vi "Config Database Top level.vi"(8 "error in (no error)":errorcluster) -> (0 "error out":errorcluster)   [LabVIEW 2013, in "ConfigDBLib.lvlib"]
doc: "Config Database is used to update the balance after Deposit, Withdrawal and Fast Casg $ 50 and Maintain the account info."
uses:
  ConfigDBLib.lvlib
  Private Controls/Queue Driver Control_Config DB.ctl
  Private Controls/Balance Update.ctl
  MainVI/TopLevelController/ToplevelControllerLibrary.lvlib
panel:
  # "Config Database is used to update the balance after Deposit, Withdrawal and Fast Casg $ 50 and Maintain the account info."
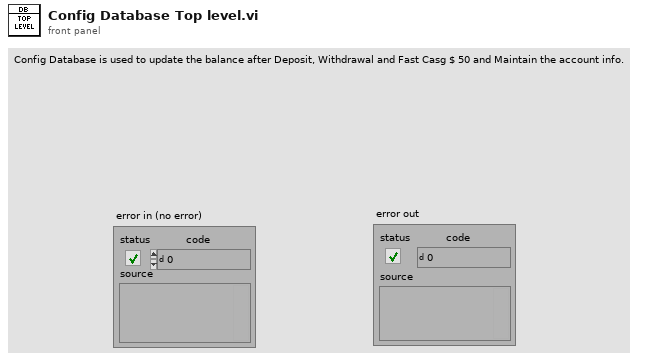
[diagram p1: front panel]
types:
  T1 = enum16{"Create Event", "Generate Event", "Destroy Event"}
  T2 = typedef "ConfigDBLib.lvlib/Queue Driver Control_Config DB.ctl" = enum16{"Init", "Enqueue", "Dequeue", "ReleaseQueue", "Exit"}
  T3 = typedef "ConfigDBLib.lvlib/Balance Update.ctl" = enum16{"Balance", "Deposit", "Withdrawal", "FastCash"}
  T4 = enum16{"Init", "Enqueue", "Dequeue", "ReleaseQueue", "Exit"}
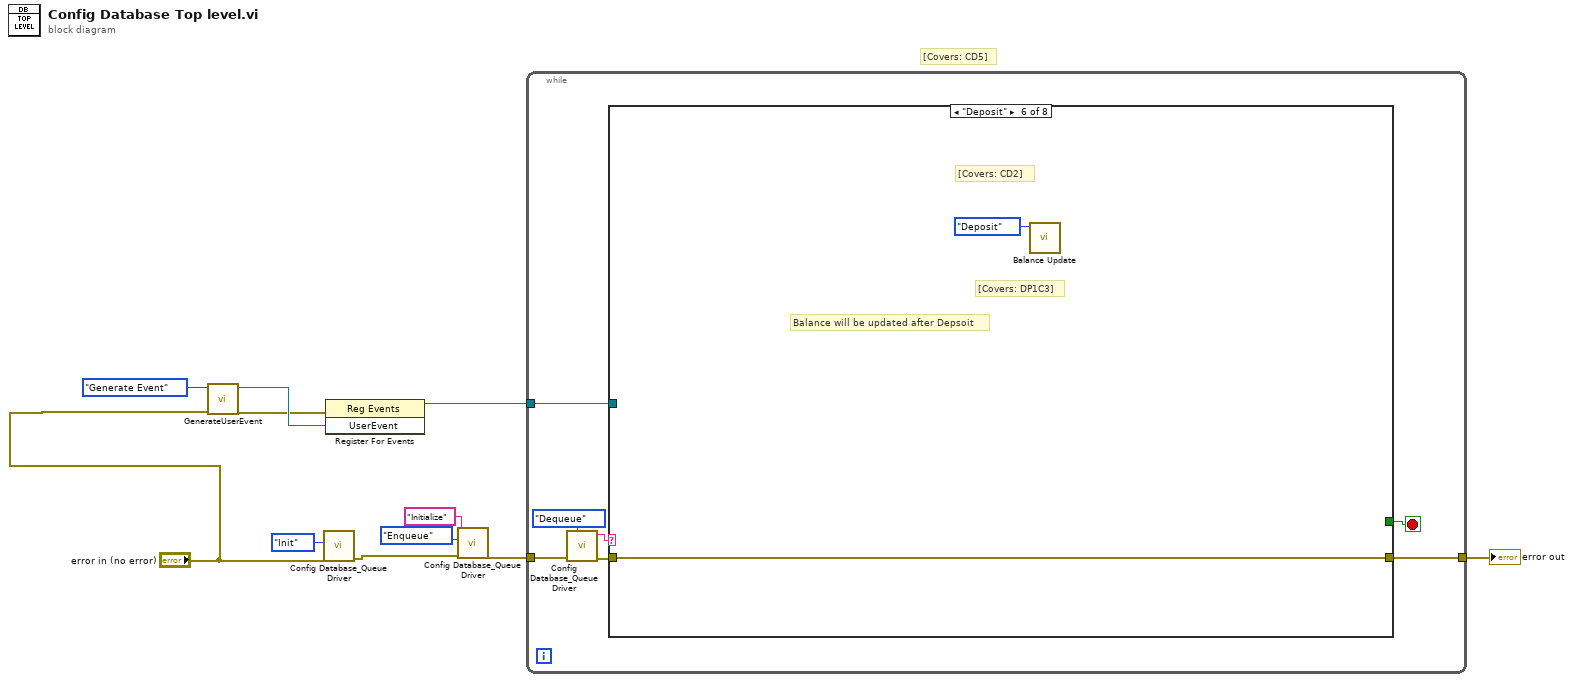
[diagram p0: block diagram]
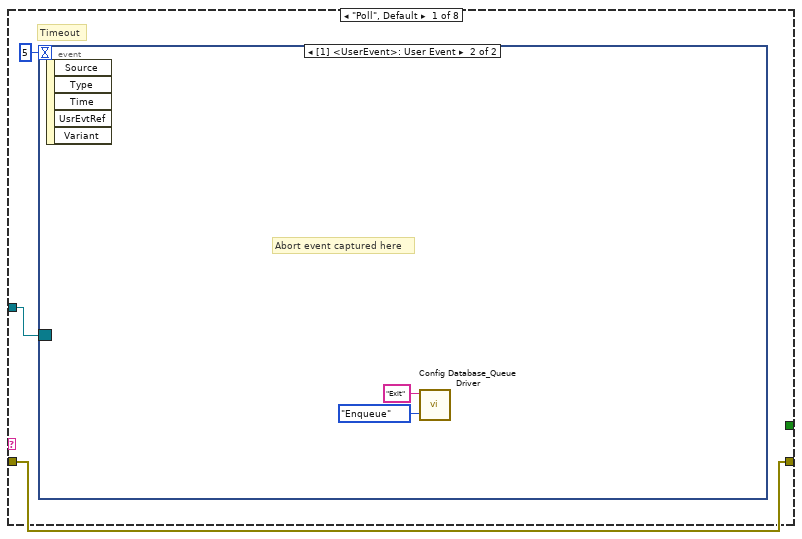
[diagram p2: hidden frame]
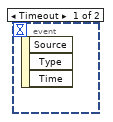
[diagram p3: hidden frame]
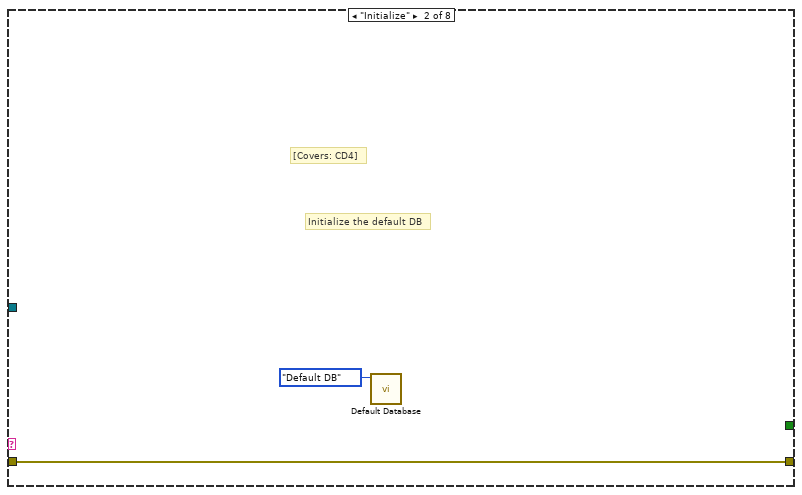
[diagram p4: hidden frame]
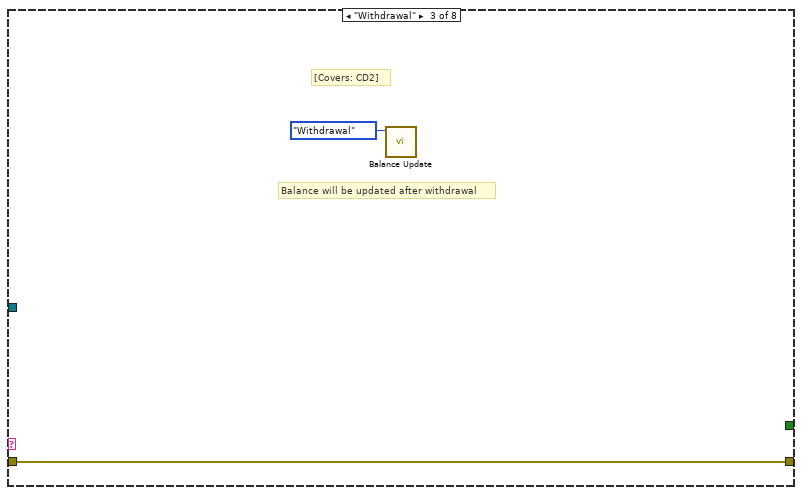
[diagram p5: hidden frame]
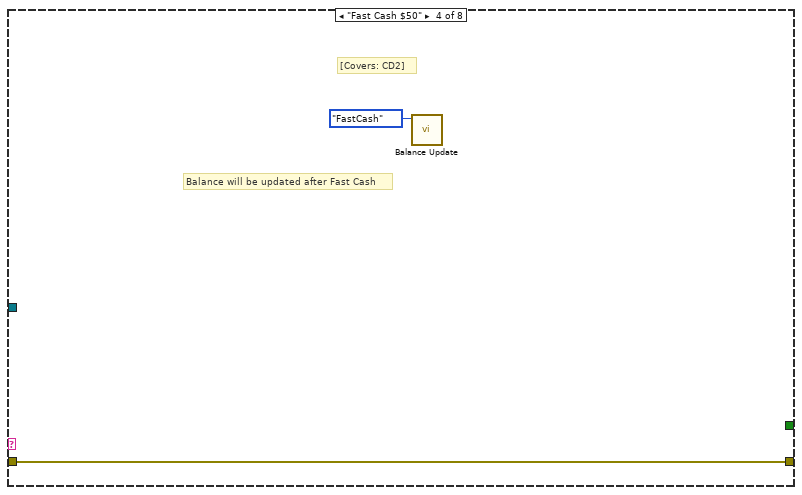
[diagram p6: hidden frame]
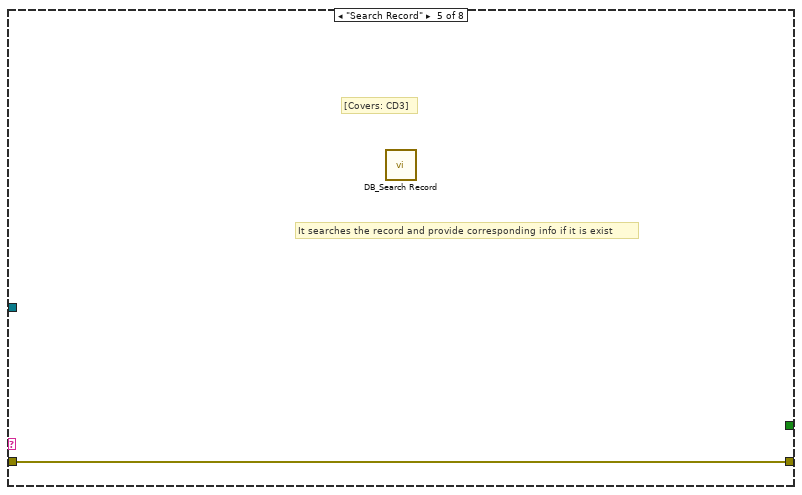
[diagram p7: hidden frame]
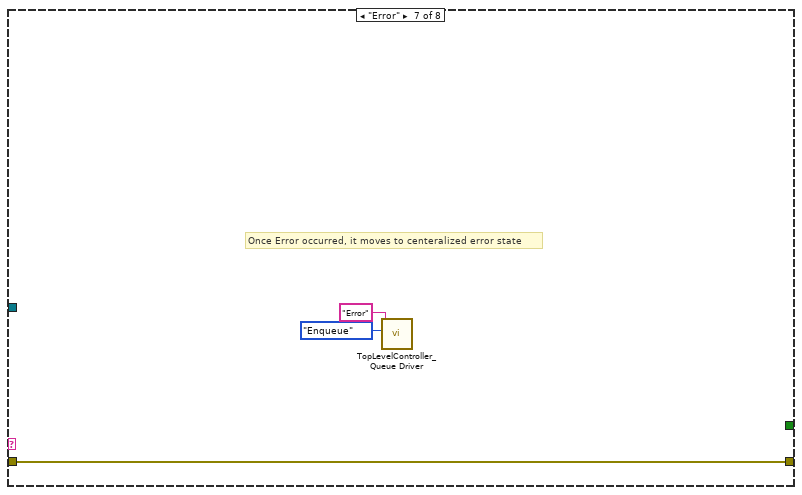
[diagram p8: hidden frame]
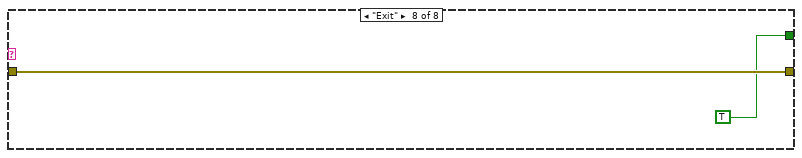
[diagram p9: hidden frame]
diagram:
  # "[Covers: CD5]"
  n1 = call "GenerateUserEvent.vi"("error in (no error)"="error in (no error)", "Event Actions"=T1."Generate Event") -> ("error out"=w3:errorcluster, "UserEvent"=w4:refnum<user-event>)  [unwired: 8 in]
  n2 = call "Config Database_Queue Driver.vi"("error in (no error)"="error in (no error)", "Enum"=Queue_Driver_Control_Config_DB."Init") -> ("error out"=w8:errorcluster)  [unwired: 8 in, 1 out]
  n3 = register-events(error in=w3, w4) -> (reference out=w2:refnum<event-registration>)  [unwired: 1 in, 1 out]
  n4 = call "Config Database_Queue Driver.vi"("error in (no error)"=w8, "Enum"=Queue_Driver_Control_Config_DB."Enqueue", "EnQ"="Initialize") -> ("error out"=w7:errorcluster)  [unwired: 7 in, 1 out]
  n5 = while {
    tunnel: w7 -> [w16]
    tunnel: [w18] -> w11
    tunnel: w2 -> [w12]
    stop <- w17 stop-if-true
    n6 = call "Config Database_Queue Driver.vi"("error in (no error)"=w16, "Enum"=Queue_Driver_Control_Config_DB."Dequeue") -> ("error out"=w13:errorcluster, "DeQ"=w14:string)  [unwired: 8 in]
    n7 = case shown="\"Deposit\"" w14 {
      tunnel: [w20 w25 w27 w29 w30 w32 w35 w37] -> w18
      tunnel: w13 -> [w20 w25 w27 w29 w30 w32 w35 w37]
      tunnel: [_ _ _ _ _ _ _ TRUE] -> w17
      tunnel: w12 -> [w19 _ _ _ _ _ _ _]
      frame "Poll", Default {
        # "Timeout"
        n8 = event shown="[1] <UserEvent>: User Event" {
          selector: w19 -> [_ _]
          dyn-events: _ -> [_ _]
          timeout: 5 -> [_ _]
          event Timeout {
            n9 = event-data() -> ()  [unwired: 1 in, 3 out]
          }
          event User Event {
            # "Abort event captured here"
            n10 = event-data() -> ()  [unwired: 1 in, 5 out]
            n11 = call "Config Database_Queue Driver.vi"("Enum"=Queue_Driver_Control_Config_DB."Enqueue", "EnQ"="Exit") -> ()  [unwired: 8 in, 2 out]
          }
        }
      }
      frame "Initialize" {
        # "Initialize the default DB"
        # "[Covers: CD4]"
        n12 = call "Default Database.vi"("Enum"=enum16{"", "Default DB", "Actual DB"}."Default DB") -> ()  [unwired: 10 in, 1 out]
      }
      frame "Withdrawal" {
        # "Balance will be updated after withdrawal"
        # "[Covers: CD2]"
        n13 = call "Balance Update.vi"("Bal.Update"=Balance_Update."Withdrawal") -> ()  [unwired: 10 in, 1 out]
      }
      frame "Fast Cash $50" {
        # "Balance will be updated after Fast Cash"
        # "[Covers: CD2]"
        n14 = call "Balance Update.vi"("Bal.Update"=Balance_Update."FastCash") -> ()  [unwired: 10 in, 1 out]
      }
      frame "Search Record" {
        # "It searches the record and provide corresponding info if it is exist"
        # "[Covers: CD3]"
        n15 = call "DB_Search Record.vi"() -> ()  [unwired: 12 in]
      }
      frame "Deposit" {
        # "Balance will be updated after Depsoit"
        # "[Covers: DP1C3]"
        # "[Covers: CD2]"
        n16 = call "Balance Update.vi"("Bal.Update"=Balance_Update."Deposit") -> ()  [unwired: 10 in, 1 out]
      }
      frame "Error" {
        # "Once Error occurred, it moves to centeralized error state"
        n17 = call "TopLevelController_Queue Driver.vi"("Enum"=T4."Enqueue", "EnQ"="Error") -> ()  [unwired: 8 in, 2 out]
      }
      frame "Exit" {
      }
    }
  }
  "error out" <- w11
